vi "Field Draw Field(Quadrada).vi"(6 "Lado,radius, stretch":i32[](array[numeric]), 8 "new picture in":picture, 9 "Offset":cluster{"Width":dbl, "Height":dbl}, 10 "Scale":dbl, 11 "Field Size":T2) -> (0 "new picture out":picture, 1 "Offset Out":cluster{"Width":dbl, "Height":dbl}, 2 "Scale Out":dbl)   [LabVIEW 2017]
panel:
  in  "left":i16=1
  in  "rect":T1
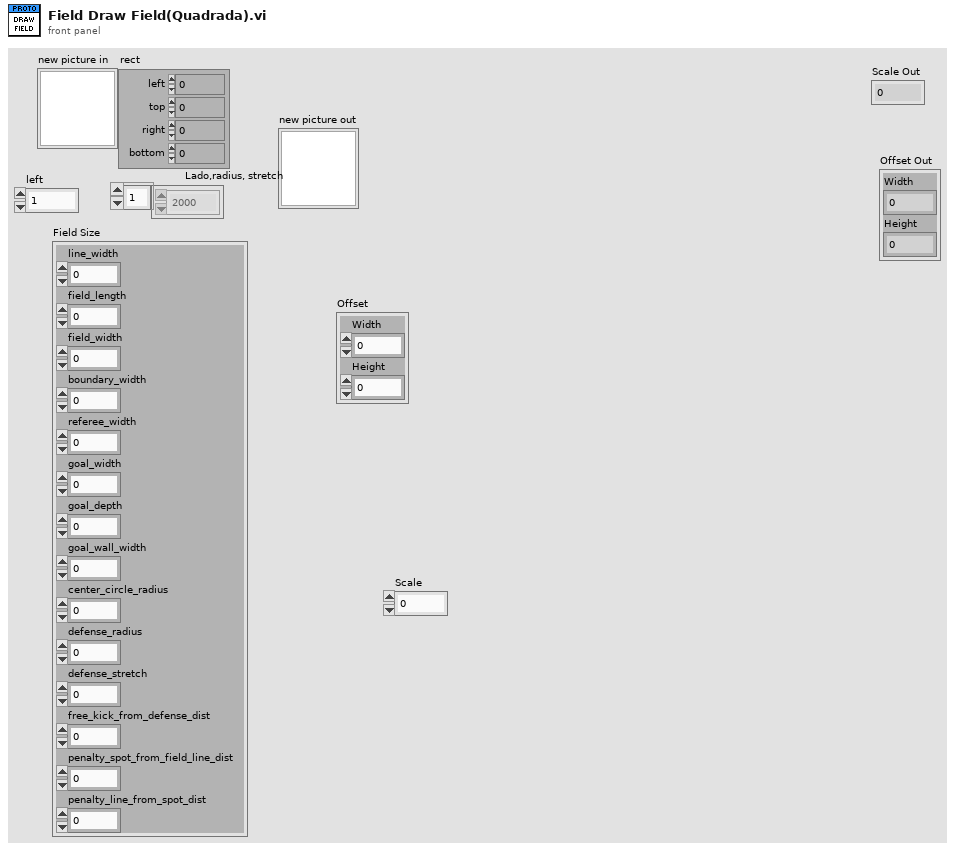
[diagram p1: front panel]
types:
  T1 = cluster{"left":i16, "top":i16, "right":i16, "bottom":i16}
  T2 = cluster{"line_width":u32, "field_length":u32, "field_width":u32, "boundary_width":u32, "referee_width":u32, "goal_width":u32, "goal_depth":u32, "goal_wall_width":u32, "center_circle_radius":u32, "defense_radius":u32, "defense_stretch":u32, "free_kick_from_defense_dist":u32, "penalty_spot_from_field_line_dist":u32, "penalty_line_from_spot_dist":u32}
  T3 = cluster{"Width":i16, "Style":enum32{"Solid", "Dash", "Dot", "DashDot", "DashDotDot"}}
  T4 = cluster{"line_width":dbl, "field_length":dbl, "field_width":dbl, "boundary_width":dbl, "referee_width":dbl, "goal_width":dbl, "goal_depth":dbl, "goal_wall_width":dbl, "center_circle_radius":dbl, "defense_radius":dbl, "defense_stretch":dbl, "free_kick_from_defense_dist":dbl, "penalty_spot_from_field_line_dist":dbl, "penalty_line_from_spot_dist":dbl}
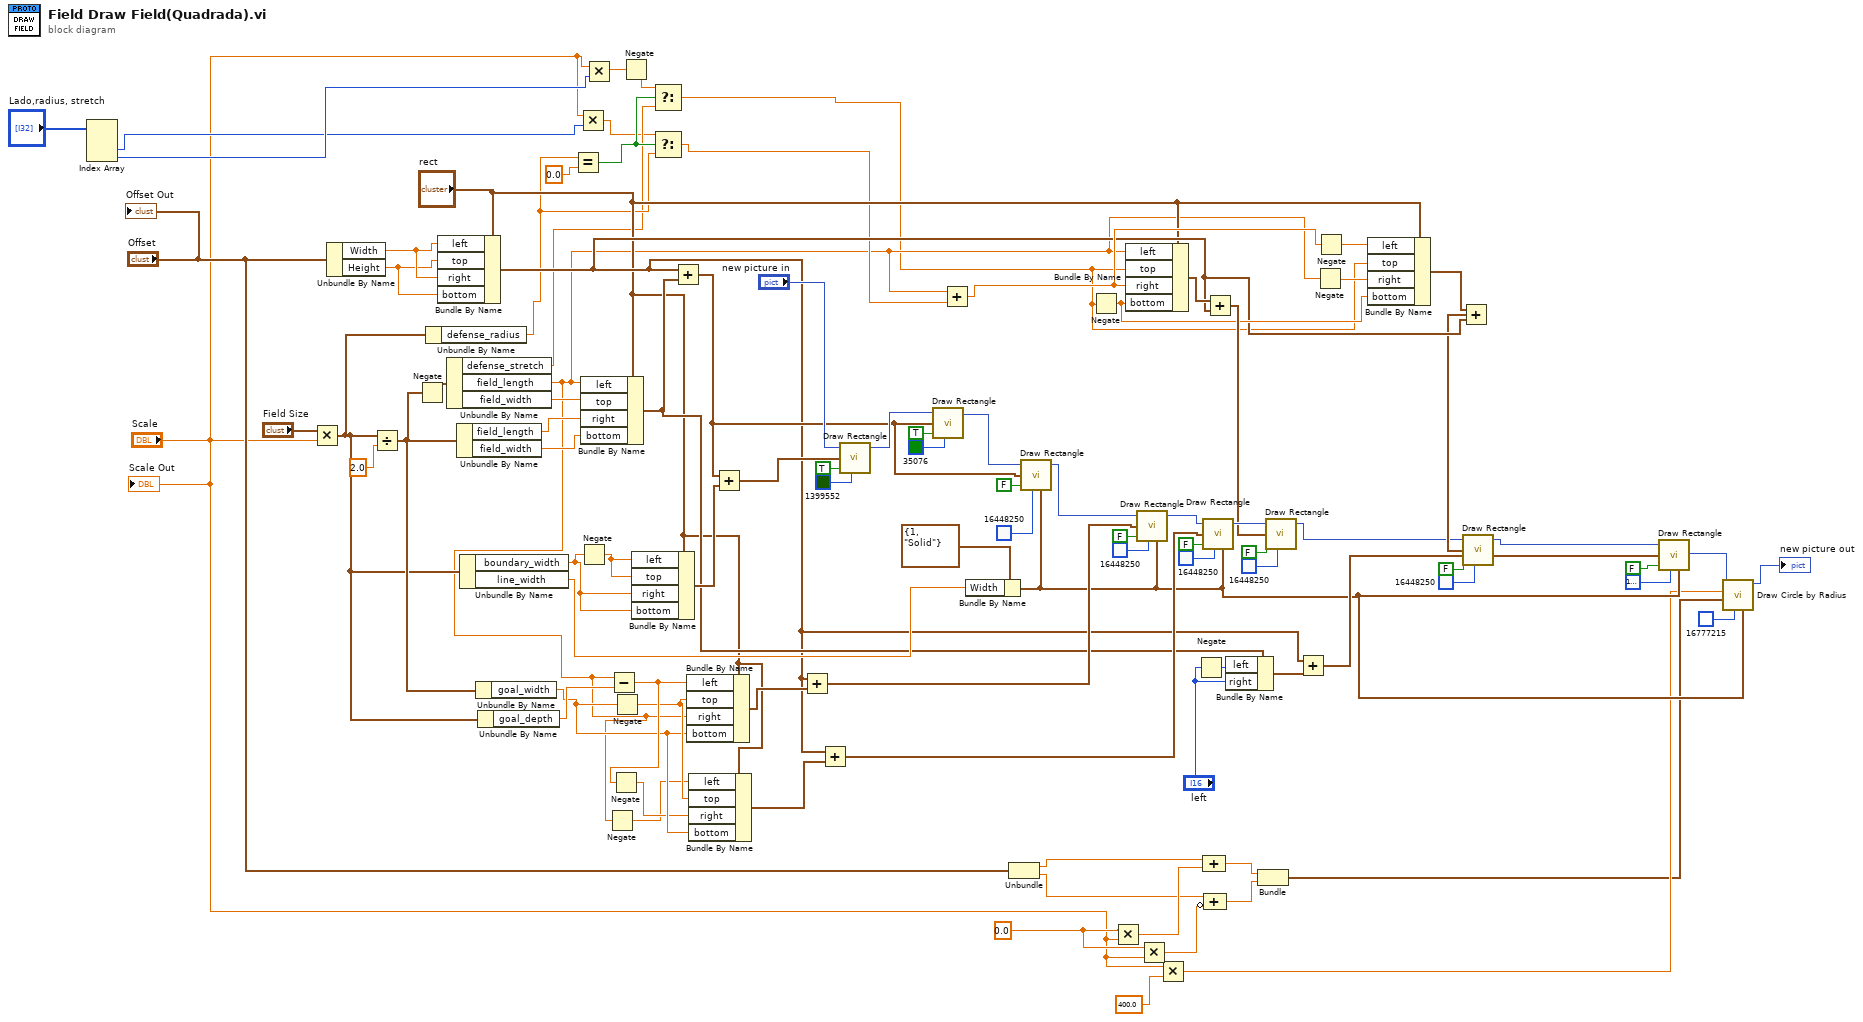
[diagram p0: block diagram]
diagram:
  w35 = 0.0 ("x")
  n1 = Index Array(array="Lado,radius, stretch") -> (element #2=w10:i32, element #3=w11:i32)  [unwired: 3 in, 1 out]
  n2 = Multiply(x="Field Size", y="Scale") -> (x*y=w34:T4)
  n3 = Unbundle By Name("Offset") -> ("Width"=w92:dbl, "Height"=w91:dbl)
  n4 = Divide(x=w34, y=2.0) -> (x/y=w67:T4)
  n5 = Negate(x=w67) -> (-x=w87:T4)
  n6 = Unbundle By Name(w34) -> ("defense_radius"=w14:dbl)
  n7 = Bundle By Name(cluster="rect", "left"=w92, "top"=w91, "right"=w92, "bottom"=w91) -> (w20:T1)
  n8 = Unbundle By Name(w87) -> ("defense_stretch"=w12:dbl, "field_length"=w6:dbl, "field_width"=w90:dbl)
  n9 = Unbundle By Name(w67) -> ("field_length"=w89:dbl, "field_width"=w88:dbl)
  n10 = Unbundle By Name(w34) -> ("boundary_width"=w85:dbl, "line_width"=w74:dbl)
  n11 = Unbundle By Name(w67) -> ("goal_width"=w61:dbl)
  n12 = Unbundle By Name(w34) -> ("goal_depth"=w66:dbl)
  n13 = Equal?(x=w14, y=0.0) -> (x = y?=w13:bool)
  n14 = Multiply(x="Scale", y=w10) -> (x*y=w8:dbl)
  n15 = Negate(x=w85) -> (-x=w86:dbl)
  n16 = Bundle By Name(cluster="rect", "left"=w6, "top"=w90, "right"=w89, "bottom"=w88) -> (w54:T1)
  n17 = Multiply(x="Scale", y=w11) -> (x*y=w4:dbl)
  n18 = Negate(x=w6) -> (-x=w57:dbl)
  n19 = Subtract(x=w6, y=w66) -> (x-y=w63:dbl)
  n20 = Negate(x=w63) -> (-x=w58:dbl)
  n21 = Negate(x=w61) -> (-x=w62:dbl)
  n22 = Negate(x=w4) -> (-x=w3:dbl)
  n23 = Bundle By Name(cluster="rect", "left"=w86, "top"=w86, "right"=w85, "bottom"=w85) -> (w84:T1)
  n24 = Select(t=w3, s=w13, f=w12) -> (s? t:f=w5:dbl)
  n25 = Select(t=w8, s=w13, f=w14) -> (s? t:f=w7:dbl)
  n26 = Add(x=w20, y=w54) -> (x+y=w45:T1)
  n27 = Bundle By Name(cluster="rect", "left"=w63, "top"=w62, "right"=w6, "bottom"=w61) -> (w65:T1)
  n28 = Bundle By Name(cluster="rect", "left"=w57, "top"=w62, "right"=w58, "bottom"=w61) -> (w60:T1)
  n29 = Add(x=w45, y=w84) -> (x+y=w80:T1)
  n30 = Add(x=w20, y=w65) -> (x+y=w64:T1)
  n31 = Add(x=w20, y=w60) -> (x+y=w59:T1)
  n32 = call <vilib>:"Draw Rectangle.vi"("picture"="new picture in", "rect"=w80, "fill?(F)"=TRUE, "color(black)"=u32 1399552) -> ("new picture"=w79:picture)  [unwired: 5 in]
  n33 = call <vilib>:"Draw Rectangle.vi"("picture"=w79, "rect"=w45, "fill?(F)"=TRUE, "color(black)"=u32 35076) -> ("new picture"=w76:picture)  [unwired: 5 in]
  n34 = Add(x=w6, y=w7) -> (x+y=w26:dbl)
  n35 = Bundle By Name(cluster=T3 {"Width"=1, "Style"=enum."Solid"} ("pen"), "Width"=w74) -> (w47:T3)
  n36 = Unbundle("Offset") -> ("Width"=w43:dbl, "Height"=w40:dbl)
  n37 = call <vilib>:"Draw Rectangle.vi"("picture"=w76, "rect"=w45, "fill?(F)"=FALSE, "color(black)"=u32 16448250, "pen"=w47) -> ("new picture"=w71:picture)  [unwired: 4 in]
  n38 = Negate(x=w5) -> (-x=w24:dbl)
  n39 = Multiply(x=w35, y="Scale") -> (x*y=w42:dbl)
  n40 = Bundle By Name(cluster="rect", "left"=w6, "top"=w5, "right"=w26, "bottom"=w24) -> (w30:T1)
  n41 = call <vilib>:"Draw Rectangle.vi"("picture"=w71, "rect"=w64, "fill?(F)"=FALSE, "color(black)"=u32 16448250, "pen"=w47) -> ("new picture"=w68:picture)  [unwired: 4 in]
  n42 = Multiply(x=w35, y="Scale") -> (x*y=w39:dbl)
  n43 = Multiply(x="Scale", y=sgl 400.0 ("radius")) -> (x*y=w37:dbl)
  n44 = Negate(x="left") -> (-x=w50:i16)
  n45 = call <vilib>:"Draw Rectangle.vi"("picture"=w68, "rect"=w59, "fill?(F)"=FALSE, "color(black)"=u32 16448250, "pen"=w47) -> ("new picture"=w31:picture)  [unwired: 4 in]
  n46 = Compound Arithmetic op=ADD(w43, w42) -> (w41:dbl)
  n47 = Compound Arithmetic op=ADD(w40, invert w39) -> (w38:dbl)
  n48 = Add(x=w30, y=w20) -> (x+y=w29:T1)
  n49 = Bundle By Name(cluster=w54, "left"=w50, "right"="left") -> (w53:T1)
  n50 = Bundle(w41, w38) -> (w36:cluster{dbl, dbl})  [unwired: 1 in]
  n51 = call <vilib>:"Draw Rectangle.vi"("picture"=w31, "rect"=w29, "fill?(F)"=FALSE, "color(black)"=u32 16448250) -> ("new picture"=w2:picture)  [unwired: 5 in]
  n52 = Add(x=w20, y=w53) -> (x+y=w52:T1)
  n53 = Negate(x=w6) -> (-x=w27:dbl)
  n54 = Negate(x=w26) -> (-x=w25:dbl)
  n55 = Bundle By Name(cluster="rect", "left"=w25, "top"=w5, "right"=w27, "bottom"=w24) -> (w21:T1)
  n56 = Add(x=w21, y=w20) -> (x+y=w19:T1)
  n57 = call <vilib>:"Draw Rectangle.vi"("picture"=w2, "rect"=w19, "fill?(F)"=FALSE, "color(black)"=u32 16448250) -> ("new picture"=w1:picture)  [unwired: 5 in]
  n58 = call <vilib>:"Draw Rectangle.vi"("picture"=w1, "rect"=w52, "fill?(F)"=FALSE, "color(black)"=u32 16777226, "pen"=w47) -> ("new picture"=w49:picture)  [unwired: 4 in]
  n59 = call <vilib>:"Draw Circle by Radius.vi"("pen"=w47, "color(black)"=u32 16777215, "pixel center"=w36, "radius"=w37, "picture"=w49) -> ("new picture"=→"new picture out":picture)  [unwired: 6 in]
  "Scale Out" <- "Scale"
  "Offset Out" <- "Offset"
